vi "Tear Down - delete root temp.vi"(8 "error in (no error)":errorcluster, 11 "tempRoot":path) -> (0 "error out":errorcluster)   [LabVIEW 2026, in "Tests.lvlib"]
doc: "Recursively deletes the temporary root created by SetUp so no test leaves artifacts behind. Runs regardless of incoming error (clears it first, mirroring Logger's \"After File Logging\"), then reports only a deletion failure. Fixture, not a test."
uses:
  Tests.lvlib
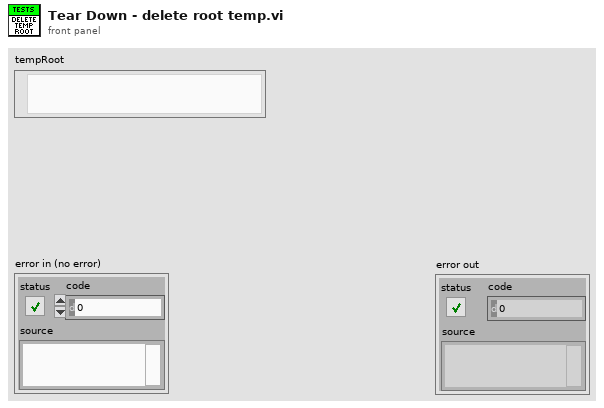
[diagram p1: front panel]
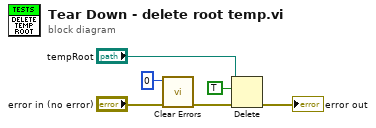
[diagram p0: block diagram]
diagram:
  n1 = call <vilib>:"Clear Errors.vi"("error in (no error)"="error in (no error)", "specific error code to clear (0: all)"=0) -> ("error out"=w4:errorcluster)  [unwired: 4 in, 1 out]
  n2 = Delete(path (use dialog)="tempRoot", entire hierarchy (F)=TRUE, error in=w4) -> (error out=→"error out":errorcluster)  [unwired: 2 in, 2 out]
